vi "Draw Trajectory.vi"(7 "Robot Index":i32, 8 "Hide Path":bool, 9 "new picture in":picture, 10 "Trajectory Data":T2(array[cluster]), 11 "Picture in":refnum<vi>) -> (0 "Path Points":cluster{"x":dbl, "y":dbl}[](array[cluster]), 2 "Output Point":T3, 3 "new picture":picture)   [LabVIEW 2025]
uses:
  Types/Segment Type.ctl
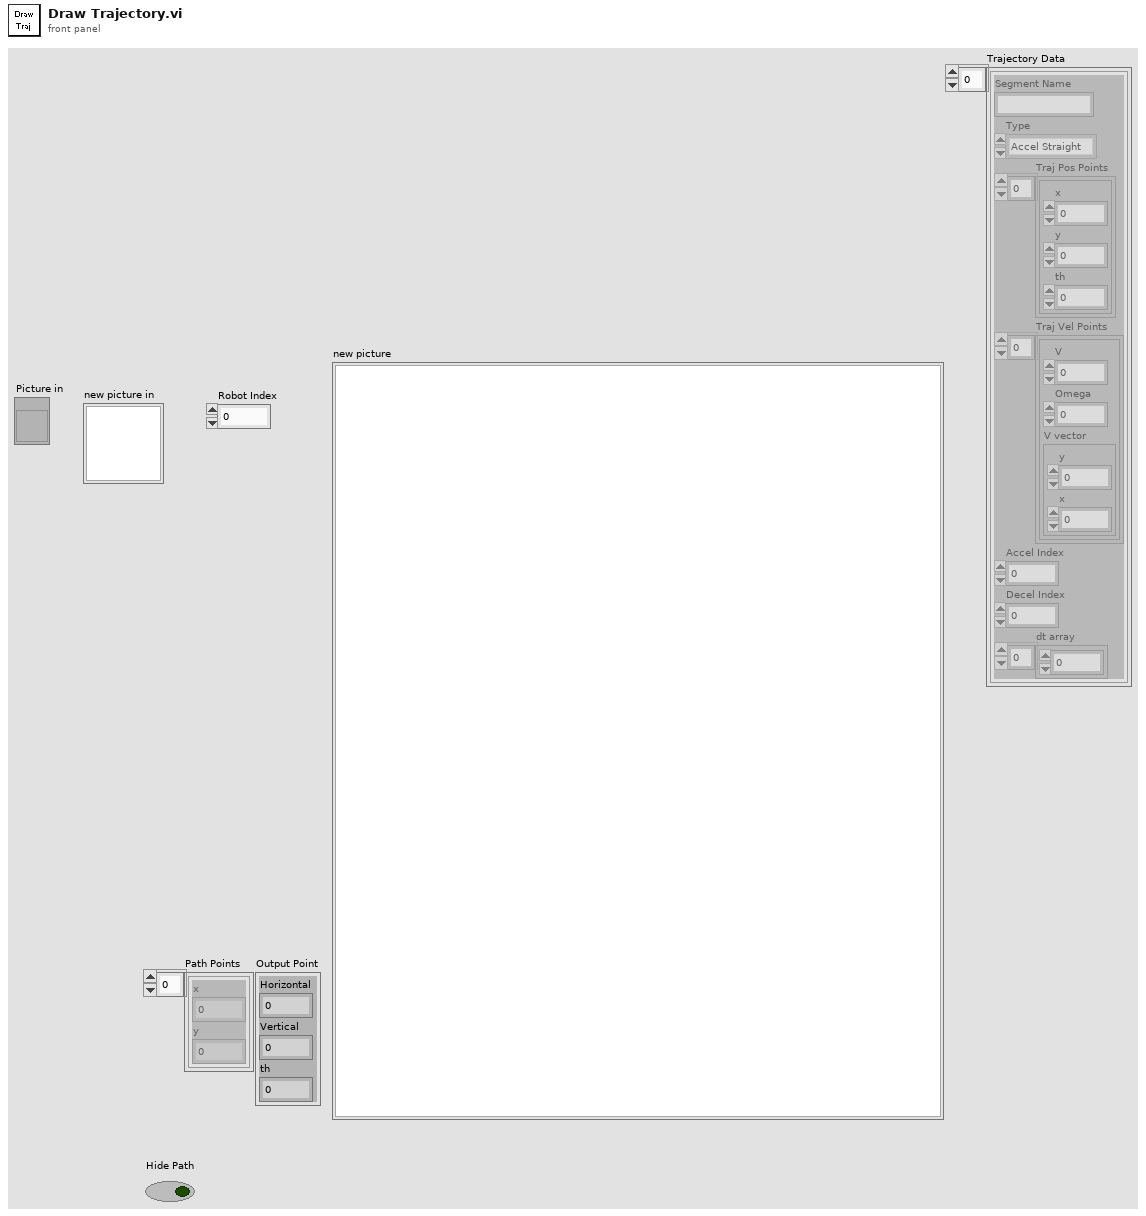
[diagram p1: front panel]
types:
  T1 = typedef "Segment Type.ctl" = enum16{"Accel Straight", "Const Straight", "Blend", "Circle", "Bezier", "Choreo"}
  T2 = cluster{"Segment Name":string, "Type":T1, "Traj Pos Points":cluster{"x":dbl, "y":dbl, "th":dbl}[], "Traj Vel Points":cluster{"V":dbl, "Omega":dbl, "V vector":cluster{"y":dbl, "x":dbl}}[], "Accel Index":i32, "Decel Index":i32, "dt array":dbl[]}[]
  T3 = cluster{"Horizontal":dbl, "Vertical":dbl, "th":dbl}
  T4 = cluster{"Width":u16, "Style":enum32{"Solid", "Dash", "Dot", "DashDot", "DashDotDot"}}
  T5 = typedef "LVPositionTypeDef.ctl" = cluster{"Left":i32, "Top":i32}
  T6 = typedef "LVBoundsTypeDef.ctl" = cluster{"Width":u32, "Height":u32}
  T7 = cluster{"V":dbl, "Omega":dbl, "V vector":cluster{"y":dbl, "x":dbl}}[]
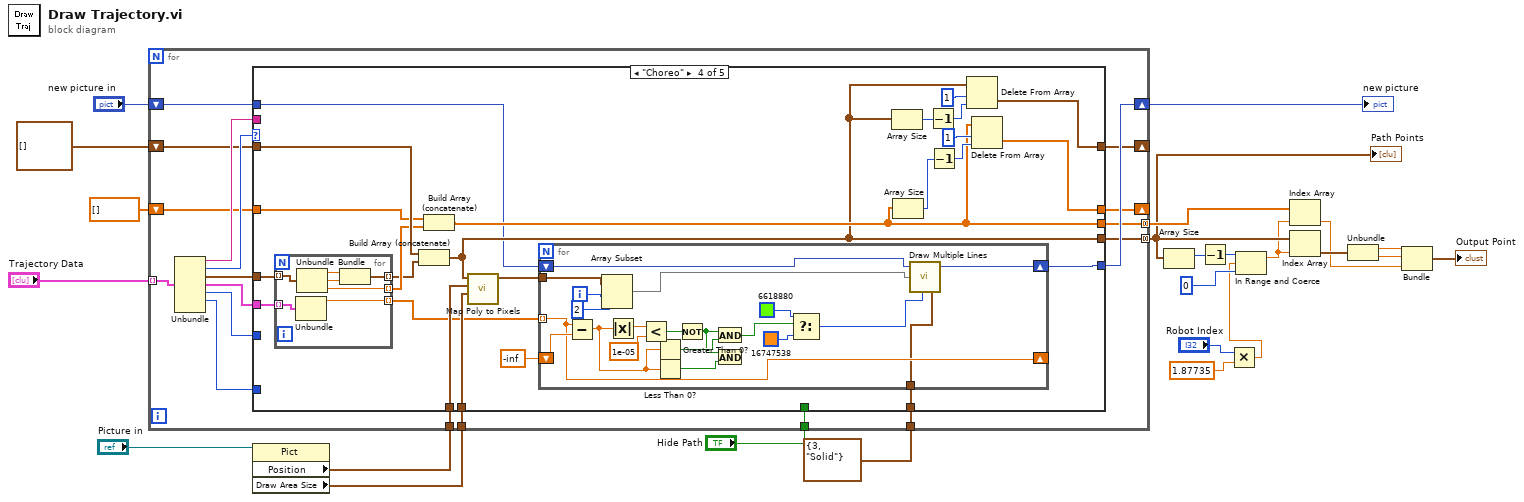
[diagram p0: block diagram]
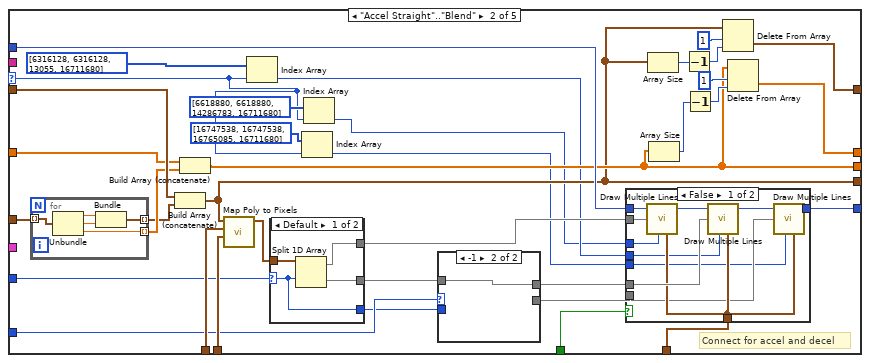
[diagram p3: hidden frame]
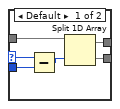
[diagram p5: hidden frame]
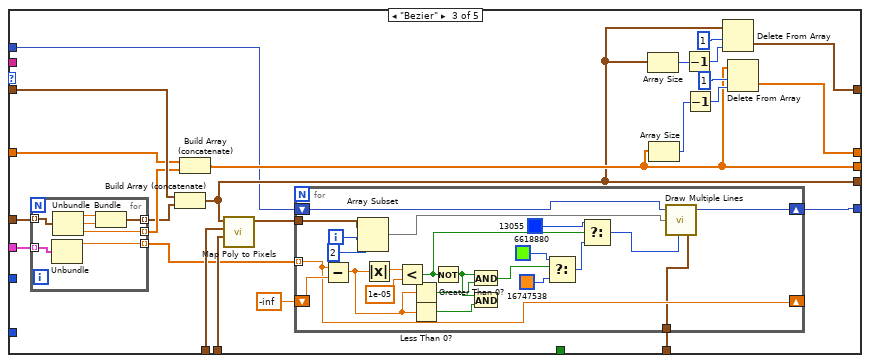
[diagram p7: hidden frame]
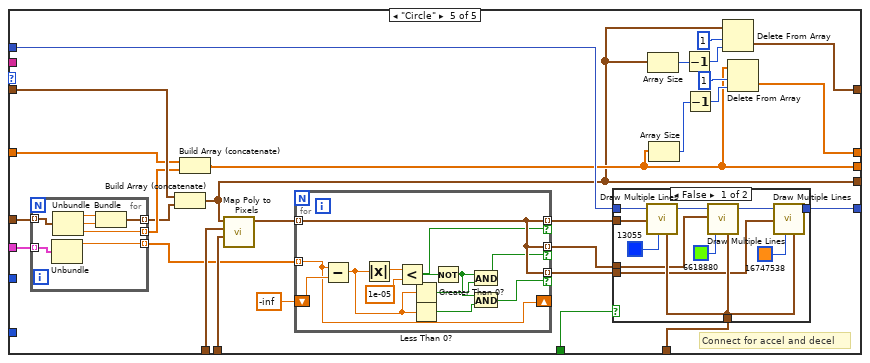
[diagram p8: hidden frame]
diagram:
  n1 = property on="Property Node" class="Pict"(reference="Picture in") -> ("Position"=w20:T5, "Draw Area Size"=w21:T6)  [unwired: 1 in, 2 out]
  n2 = for {
    tunnel: "Trajectory Data" -> [w43] mode=indexing
    shift-right: [w36] -> w19
    shift-left: "new picture in" -> [w35]
    tunnel: T4 {"Width"=3, "Style"=enum."Solid"} ("pen") -> [w39]
    tunnel: w21 -> [w38]
    tunnel: w20 -> [w37]
    tunnel: [w33] -> w12 mode=concatenating
    tunnel: [w32] -> w13 mode=concatenating
    shift-right: [w30] -> _
    shift-left: cluster{"x":dbl, "y":dbl}[] [] -> [w29]
    shift-right: [w28] -> _
    shift-left: dbl[] [] -> [w27]
    tunnel: "Hide Path" -> [w25]
    n3 = Unbundle(w43) -> ("Segment Name"=w42:string, "Type"=w34:T1, "Traj Pos Points"=w41:cluster{"x":dbl, "y":dbl, "th":dbl}[], "Traj Vel Points"=w40:T7, "Accel Index"=w31:i32, "Decel Index"=w26:i32)  [unwired: 1 out]
    n4 = case shown="\"Choreo\"" w34 {
      selector: w34 -> [_ w50 _ _ _]
      tunnel: w42 -> [_ _ _ _ _]
      tunnel: w41 -> [_ w82 w135 w188 w243]
      tunnel: w40 -> [_ _ w118 w171 w222]
      tunnel: w39 -> [_ w61 w114 w167 w226]
      tunnel: w38 -> [_ w81 w134 w187 w242]
      tunnel: w37 -> [_ w79 w133 w186 w240]
      tunnel: [w46 w62 w112 w165 w227] -> w36
      tunnel: w35 -> [w46 w80 w113 w166 w241]
      tunnel: [_ w56 w119 w172 w224] -> w33
      tunnel: [_ w68 w123 w176 w230] -> w32
      tunnel: w31 -> [_ w65 _ _ _]
      tunnel: [w45 w73 w128 w181 w235] -> w30
      tunnel: w29 -> [w45 w76 w131 w184 w238]
      tunnel: [w44 w69 w124 w177 w231] -> w28
      tunnel: w27 -> [w44 w66 w121 w174 w228]
      tunnel: w26 -> [_ w64 _ _ _]
      tunnel: w25 -> [_ w47 _ _ w223]
      frame Default {
      }
      frame "Accel Straight".."Blend" {
        # "Connect for accel and decel"
        n5 = for {
          tunnel: w82 -> [w111] mode=indexing
          tunnel: [w110] -> w57 mode=indexing
          tunnel: [w107] -> w67 mode=indexing
          n6 = Unbundle(w111) -> ("x"=w109:dbl, "y"=w108:dbl, "th"=w107:dbl)
          n7 = Bundle("x"=w109, "y"=w108) -> (w110:cluster{"x":dbl, "y":dbl})  [unwired: 1 in]
        }
        n8 = Build Array (concatenate)(w76, w57) -> (w56:cluster{"x":dbl, "y":dbl}[])
        n9 = Build Array (concatenate)(w66, w67) -> (w68:dbl[])
        n10 = call "Map Poly to Pixels.vi"("Draw Area Size"=w81, "Position"=w79, "Coords"=w56) -> ("Coords"=w55:cluster{"Horizontal":dbl, "Vertical":dbl}[])  [unwired: 8 in]
        n11 = Index Array(array=u32[] [6316128, 6316128, 13055, 16711680], index=w50) -> (element=w53:u32)
        n12 = case shown="Default" w65 {
          selector: w65 -> [w102 _]
          tunnel: w55 -> [w105 w106]
          tunnel: [w103 _] -> w54
          tunnel: [w104 w106] -> w59
          tunnel: [w102 _] -> w58
          frame Default {
            n13 = Split 1D Array(array=w105, index=w102) -> (first subarray=w103:cluster{"Horizontal":dbl, "Vertical":dbl}[], second subarray=w104:cluster{"Horizontal":dbl, "Vertical":dbl}[])
          }
          frame -1 {
          }
        }
        n14 = Index Array(array=u32[] [16747538, 16747538, 16765085, 16711680], index=w50) -> (element=w48:u32)
        n15 = Index Array(array=u32[] [6618880, 6618880, 14286783, 16711680], index=w50) -> (element=w49:u32)
        n16 = case shown="-1" w64 {
          selector: w64 -> [w97 _]
          tunnel: w59 -> [w100 w101]
          tunnel: [w99 w101] -> w63
          tunnel: [w98 _] -> w60
          tunnel: w58 -> [w96 _]
          frame Default {
            n17 = Subtract(x=w97, y=w96) -> (x-y=w95:i32)
            n18 = Split 1D Array(array=w100, index=w95) -> (first subarray=w99:cluster{"Horizontal":dbl, "Vertical":dbl}[], second subarray=w98:cluster{"Horizontal":dbl, "Vertical":dbl}[])
          }
          frame -1 {
          }
        }
        n19 = case shown="False" w47 {
          tunnel: w80 -> [w93 w94]
          tunnel: w63 -> [w91 _]
          tunnel: [w89 w94] -> w62
          tunnel: w61 -> [w88 _]
          tunnel: w60 -> [w87 _]
          tunnel: w54 -> [w86 _]
          tunnel: w53 -> [w85 _]
          tunnel: w49 -> [w84 _]
          tunnel: w48 -> [w83 _]
          frame False {
            n20 = call <vilib>:"Draw Multiple Lines.vi"("picture"=w93, "line endpoints"=w86, "color(black)"=w84, "pen"=w88) -> ("new picture"=w92:picture)  [unwired: 5 in]
            n21 = call <vilib>:"Draw Multiple Lines.vi"("picture"=w92, "line endpoints"=w91, "color(black)"=w85, "pen"=w88) -> ("new picture"=w90:picture)  [unwired: 5 in]
            n22 = call <vilib>:"Draw Multiple Lines.vi"("picture"=w90, "line endpoints"=w87, "color(black)"=w83, "pen"=w88) -> ("new picture"=w89:picture)  [unwired: 5 in]
          }
          frame True {
          }
        }
        n23 = Array Size(array=w56) -> (size(s)=w77:i32)
        n24 = Array Size(array=w68) -> (size(s)=w70:i32)
        n25 = Decrement(x=w77) -> (x-1=w74:i32)
        n26 = Decrement(x=w70) -> (x-1=w72:i32)
        n27 = Delete From Array(array=w56, length=1, index=w74) -> (deleted portion=w73:cluster{"x":dbl, "y":dbl}[])  [unwired: 1 out]
        n28 = Delete From Array(array=w68, length=1, index=w72) -> (deleted portion=w69:dbl[])  [unwired: 1 out]
      }
      frame "Bezier" {
        n29 = for {
          tunnel: w135 -> [w164] mode=indexing
          tunnel: [w163] -> w120 mode=indexing
          tunnel: [w160] -> w122 mode=indexing
          tunnel: w118 -> [w159] mode=indexing
          tunnel: [w158] -> w116 mode=indexing
          n30 = Unbundle(w159) -> ("V"=w158:dbl)  [unwired: 2 out]
          n31 = Unbundle(w164) -> ("x"=w162:dbl, "y"=w161:dbl, "th"=w160:dbl)
          n32 = Bundle("x"=w162, "y"=w161) -> (w163:cluster{"x":dbl, "y":dbl})  [unwired: 1 in]
        }
        n33 = Build Array (concatenate)(w131, w120) -> (w119:cluster{"x":dbl, "y":dbl}[])
        n34 = Build Array (concatenate)(w121, w122) -> (w123:dbl[])
        n35 = call "Map Poly to Pixels.vi"("Draw Area Size"=w134, "Position"=w133, "Coords"=w119) -> ("Coords"=w117:cluster{"Horizontal":dbl, "Vertical":dbl}[])  [unwired: 8 in]
        n36 = for {
          tunnel: w117 -> [w137]
          tunnel: w116 -> [w154] mode=indexing
          shift-right: [w154] -> _
          shift-left: -inf -> [w157]
          tunnel: w114 -> [w142]
          shift-right: [w140] -> w112
          shift-left: w113 -> [w141]
          i -> [w139]
          n37 = Subtract(x=w154, y=w157) -> (x-y=w152:dbl)
          n38 = Array Subset(array=w137, index=w139, length=2) -> (w136:cluster{"Horizontal":dbl, "Vertical":dbl}[])
          n39 = Absolute Value(x=w152) -> (abs(x)=w156:dbl)
          n40 = Less?(x=w156, y=1e-05) -> (x < y?=w148:bool)
          n41 = Greater Than 0?(x=w152) -> (x > 0?=w153:bool)
          n42 = Less Than 0?(x=w152) -> (x < 0?=w151:bool)
          n43 = Not(x=w148) -> (.not. x?=w150:bool)
          n44 = And(x=w150, y=w153) -> (x .and. y?=w149:bool)
          n45 = And(x=w150, y=w151) -> ()  [unwired: 1 out]
          n46 = Select(t=u32 6618880 ("color(black)"), s=w149, f=u32 16747538 ("color(black)")) -> (s? t:f=w146:u32)
          n47 = Select(t=u32 13055 ("color(black)"), s=w148, f=w146) -> (s? t:f=w143:u32)
          n48 = call <vilib>:"Draw Multiple Lines.vi"("picture"=w141, "line endpoints"=w136, "color(black)"=w143, "pen"=w142) -> ("new picture"=w140:picture)  [unwired: 5 in]
        }
        n49 = Array Size(array=w119) -> (size(s)=w132:i32)
        n50 = Array Size(array=w123) -> (size(s)=w125:i32)
        n51 = Decrement(x=w132) -> (x-1=w129:i32)
        n52 = Decrement(x=w125) -> (x-1=w127:i32)
        n53 = Delete From Array(array=w119, length=1, index=w129) -> (deleted portion=w128:cluster{"x":dbl, "y":dbl}[])  [unwired: 1 out]
        n54 = Delete From Array(array=w123, length=1, index=w127) -> (deleted portion=w124:dbl[])  [unwired: 1 out]
      }
      frame "Choreo" {
        n55 = for {
          tunnel: w188 -> [w215] mode=indexing
          tunnel: [w214] -> w173 mode=indexing
          tunnel: [w211] -> w175 mode=indexing
          tunnel: w171 -> [w210] mode=indexing
          tunnel: [w209] -> w169 mode=indexing
          n56 = Unbundle(w210) -> ("V"=w209:dbl)  [unwired: 2 out]
          n57 = Unbundle(w215) -> ("x"=w213:dbl, "y"=w212:dbl, "th"=w211:dbl)
          n58 = Bundle("x"=w213, "y"=w212) -> (w214:cluster{"x":dbl, "y":dbl})  [unwired: 1 in]
        }
        n59 = Build Array (concatenate)(w184, w173) -> (w172:cluster{"x":dbl, "y":dbl}[])
        n60 = Build Array (concatenate)(w174, w175) -> (w176:dbl[])
        n61 = call "Map Poly to Pixels.vi"("Draw Area Size"=w187, "Position"=w186, "Coords"=w172) -> ("Coords"=w170:cluster{"Horizontal":dbl, "Vertical":dbl}[])  [unwired: 8 in]
        n62 = for {
          tunnel: w170 -> [w190]
          tunnel: w169 -> [w205] mode=indexing
          shift-right: [w205] -> _
          shift-left: -inf -> [w208]
          tunnel: w167 -> [w195]
          shift-right: [w193] -> w165
          shift-left: w166 -> [w194]
          i -> [w192]
          n63 = Subtract(x=w205, y=w208) -> (x-y=w203:dbl)
          n64 = Array Subset(array=w190, index=w192, length=2) -> (w189:cluster{"Horizontal":dbl, "Vertical":dbl}[])
          n65 = Absolute Value(x=w203) -> (abs(x)=w207:dbl)
          n66 = Less?(x=w207, y=1e-05) -> (x < y?=w199:bool)
          n67 = Greater Than 0?(x=w203) -> (x > 0?=w204:bool)
          n68 = Less Than 0?(x=w203) -> (x < 0?=w202:bool)
          n69 = Not(x=w199) -> (.not. x?=w201:bool)
          n70 = And(x=w201, y=w204) -> (x .and. y?=w200:bool)
          n71 = And(x=w201, y=w202) -> ()  [unwired: 1 out]
          n72 = Select(t=u32 6618880 ("color(black)"), s=w200, f=u32 16747538 ("color(black)")) -> (s? t:f=w196:u32)
          n73 = call <vilib>:"Draw Multiple Lines.vi"("picture"=w194, "line endpoints"=w189, "color(black)"=w196, "pen"=w195) -> ("new picture"=w193:picture)  [unwired: 5 in]
        }
        n74 = Array Size(array=w172) -> (size(s)=w185:i32)
        n75 = Array Size(array=w176) -> (size(s)=w178:i32)
        n76 = Decrement(x=w185) -> (x-1=w182:i32)
        n77 = Decrement(x=w178) -> (x-1=w180:i32)
        n78 = Delete From Array(array=w172, length=1, index=w182) -> (deleted portion=w181:cluster{"x":dbl, "y":dbl}[])  [unwired: 1 out]
        n79 = Delete From Array(array=w176, length=1, index=w180) -> (deleted portion=w177:dbl[])  [unwired: 1 out]
      }
      frame "Circle" {
        # "Connect for accel and decel"
        n80 = for {
          tunnel: w243 -> [w274] mode=indexing
          tunnel: [w273] -> w225 mode=indexing
          tunnel: [w270] -> w229 mode=indexing
          tunnel: w222 -> [w269] mode=indexing
          tunnel: [w268] -> w220 mode=indexing
          n81 = Unbundle(w269) -> ("V"=w268:dbl)  [unwired: 2 out]
          n82 = Unbundle(w274) -> ("x"=w272:dbl, "y"=w271:dbl, "th"=w270:dbl)
          n83 = Bundle("x"=w272, "y"=w271) -> (w273:cluster{"x":dbl, "y":dbl})  [unwired: 1 in]
        }
        n84 = Build Array (concatenate)(w238, w225) -> (w224:cluster{"x":dbl, "y":dbl}[])
        n85 = Build Array (concatenate)(w228, w229) -> (w230:dbl[])
        n86 = call "Map Poly to Pixels.vi"("Draw Area Size"=w242, "Position"=w240, "Coords"=w224) -> ("Coords"=w221:cluster{"Horizontal":dbl, "Vertical":dbl}[])  [unwired: 8 in]
        n87 = for {
          tunnel: w221 -> [w252] mode=indexing
          tunnel: w220 -> [w251] mode=indexing
          shift-right: [w251] -> _
          shift-left: -inf -> [w255]
          tunnel: [w252] -> w218 mode=indexing if=w246
          tunnel: [w252] -> w217 mode=indexing if=w245
          tunnel: [w252] -> w216 mode=indexing if=w244
          n88 = Subtract(x=w251, y=w255) -> (x-y=w249:dbl)
          n89 = Absolute Value(x=w249) -> (abs(x)=w254:dbl)
          n90 = Less?(x=w254, y=1e-05) -> (x < y?=w246:bool)
          n91 = Greater Than 0?(x=w249) -> (x > 0?=w250:bool)
          n92 = Less Than 0?(x=w249) -> (x < 0?=w248:bool)
          n93 = Not(x=w246) -> (.not. x?=w247:bool)
          n94 = And(x=w247, y=w250) -> (x .and. y?=w245:bool)
          n95 = And(x=w247, y=w248) -> (x .and. y?=w244:bool)
        }
        n96 = case shown="False" w223 {
          tunnel: w241 -> [w266 w267]
          tunnel: [w263 w267] -> w227
          tunnel: w226 -> [w262 _]
          tunnel: w218 -> [w259 _]
          tunnel: w217 -> [w258 _]
          tunnel: w216 -> [w257 _]
          frame False {
            n97 = call <vilib>:"Draw Multiple Lines.vi"("picture"=w266, "line endpoints"=w259, "color(black)"=u32 13055, "pen"=w262) -> ("new picture"=w265:picture)  [unwired: 5 in]
            n98 = call <vilib>:"Draw Multiple Lines.vi"("picture"=w265, "line endpoints"=w258, "color(black)"=u32 6618880, "pen"=w262) -> ("new picture"=w264:picture)  [unwired: 5 in]
            n99 = call <vilib>:"Draw Multiple Lines.vi"("picture"=w264, "line endpoints"=w257, "color(black)"=u32 16747538, "pen"=w262) -> ("new picture"=w263:picture)  [unwired: 5 in]
          }
          frame True {
          }
        }
        n100 = Array Size(array=w224) -> (size(s)=w239:i32)
        n101 = Array Size(array=w230) -> (size(s)=w232:i32)
        n102 = Decrement(x=w239) -> (x-1=w236:i32)
        n103 = Decrement(x=w232) -> (x-1=w234:i32)
        n104 = Delete From Array(array=w224, length=1, index=w236) -> (deleted portion=w235:cluster{"x":dbl, "y":dbl}[])  [unwired: 1 out]
        n105 = Delete From Array(array=w230, length=1, index=w234) -> (deleted portion=w231:dbl[])  [unwired: 1 out]
      }
    }
  }
  "new picture" <- w19
  "Path Points" <- w12
  n106 = Array Size(array=w12) -> (size(s)=w11:i32)
  n107 = Decrement(x=w11) -> (x-1=w10:i32)
  n108 = Multiply(x="Robot Index", y=1.87735) -> (x*y=w1:dbl)
  n109 = In Range and Coerce(upper limit=w10, x=w1, lower limit=u16 0 ("Width")) -> (coerced(x)=w8:dbl)  [unwired: 1 out]
  n110 = Index Array(array=w13, index=w8) -> (element=w15:dbl)
  n111 = Index Array(array=w12, index=w8) -> (element=w18:cluster{"x":dbl, "y":dbl})
  n112 = Unbundle(w18) -> ("x"=w17:dbl, "y"=w16:dbl)
  n113 = Bundle("x"=w17, "y"=w16, "th"=w15) -> (→"Output Point":cluster{"x":dbl, "y":dbl, "th":dbl})  [unwired: 1 in]
